vi "Extract Doubles.vi"(4 "error in":errorcluster, 6 "String":string="values: 53k, 42M, separator 37u string as received", 7 "Eng Units?":bool) -> (0 "error out":errorcluster, 3 "Data":dbl[](array[numeric]) format="%_6e")   [LabVIEW 2020]
doc: "Finds all numbers in the given string and puts them into an array as double-precision numbers. All of the following formats are recognized:\n123 1.23 1.23e2 1.23E2\nNo spaces or other characters may appear within the number, but any characters may appear before or after the number.\nThe engineering units convers suffixes k,m,u as 1000, 0.001 and 1e-6 multipliers. Case of the units is not important which means that \"M\" is the same as \"m\" and denotes a 0.001 multiplier.\nModified from examples which did not work, by\nScott Hannahs, <sth@magnet.fsu.edu> NHMFL-FSU, May 2003"
uses:
  <userlib>/_OpenG.lib/array/array.llb/Empty 1D Array (DBL)__ogtk.vi
panel:
  # "This VI takes a string containing multiple numbers and extracts those numbers into an array.  See the Get Info dialog box for more information."
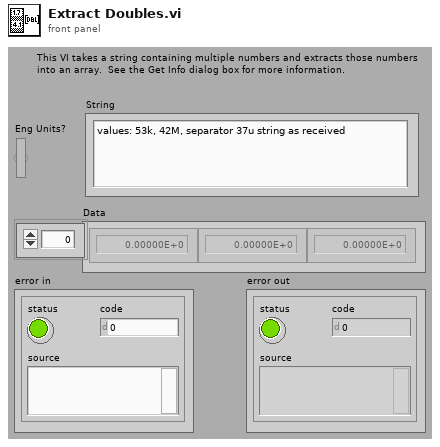
[diagram p1: front panel]
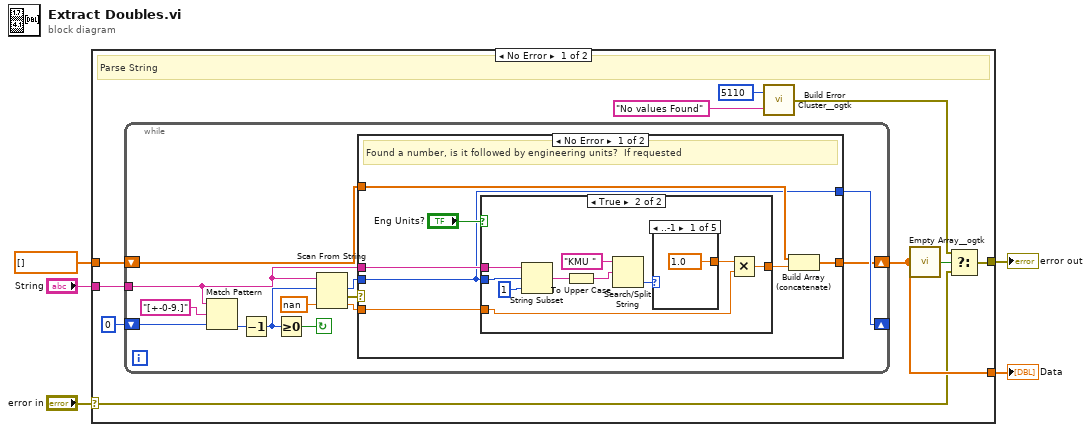
[diagram p0: block diagram]
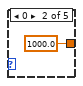
[diagram p3: hidden frame]
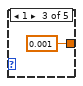
[diagram p4: hidden frame]
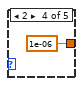
[diagram p5: hidden frame]
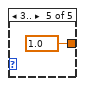
[diagram p6: hidden frame]
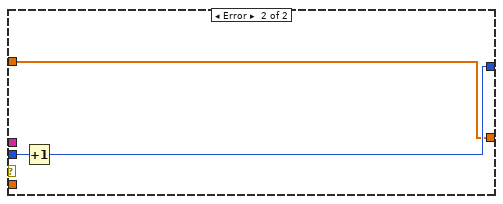
[diagram p7: hidden frame]
diagram:
  n1 = case shown="No Error" "error in" {
    selector: "error in" -> [w11 w56]
    tunnel: "String" -> [w15 _]
    tunnel: dbl[] [] ("Double Precision Array") -> [w14 w55]
    tunnel: [w12 w56] -> w2
    tunnel: [w13 w55] -> w1
    frame No Error {
      # "Parse String"
      n2 = while {
        shift-left: w14 -> [w20]
        shift-right: [w19] -> w13
        tunnel: w15 -> [w17]
        shift-left: u32 0 -> [w27]
        shift-right: [w23] -> _
        stop <- w21 continue-if-true
        n3 = Match Pattern(string=w17, regular expression="[+-0-9.]", offset (0)=w27) -> (offset past match=w26:i32)  [unwired: 3 out]
        n4 = Decrement(x=w26) -> (x-1=w25:i32)
        n5 = Greater Or Equal To 0?(x=w25) -> (x >= 0?=w21:bool)
        n6 = Scan From String(input string=w17, initial scan location=w25, default 1=nan) -> (offset past scan=w22:u32, error out=w16:errorcluster, output 1=w18:dbl)  [unwired: 2 in, 1 out]
        n7 = case shown="No Error" w16 {
          tunnel: [w29 w54] -> w23
          tunnel: w22 -> [w29 w53]
          tunnel: w20 -> [w35 w52]
          tunnel: [w34 w52] -> w19
          tunnel: w18 -> [w32 _]
          tunnel: w17 -> [w30 _]
          frame No Error {
            # "Found a number, is it followed by engineering units?  If requested"
            n8 = case shown="True" "Eng Units?" {
              tunnel: [w36 w41] -> w31
              tunnel: w32 -> [w36 w42]
              tunnel: w30 -> [_ w44]
              tunnel: w29 -> [_ w40]
              frame False {
              }
              frame True {
                n9 = String Subset(string=w44, offset (0)=w40, length (rest)=1 ("length")) -> (substring=w38:string)
                n10 = To Upper Case(1:w38) -> (0:w39:string)
                n11 = Search/Split String(string="KMU ", search string/char (-)=w39) -> (offset of match=w37:i32)  [unwired: 1 in, 2 out]
                n12 = case shown="..-1" w37 {
                  tunnel: [1.0 ("y") 1000.0 ("y") 0.001 ("y") 1e-06 ("y") 1.0 ("y")] -> w43
                  frame ..-1 {
                  }
                  frame 0 {
                  }
                  frame 1 {
                  }
                  frame 2 {
                  }
                  frame 3.. {
                  }
                }
                n13 = Multiply(x=w43, y=w42) -> (x*y=w41:dbl)
              }
            }
            n14 = Build Array (concatenate)(w35, w31) -> (w34:dbl[])
          }
          frame Error {
            n15 = Increment(x=w53) -> (x+1=w54:u32)
          }
        }
      }
      n16 = call <userlib>:"Build Error Cluster__ogtk.vi"("String to Prepend to source (\"\")"="No values Found" ("source"), "code"=5110) -> ("error out"=w8:errorcluster)
      n17 = call-poly <userlib>:"Empty Array__ogtk.vi"("Array"=w13) -> ("Empty Array?"=w10:bool)  [unwired: 8 in]
      n18 = Select(t=w8, s=w10, f=w11) -> (s? t:f=w12:errorcluster)
    }
    frame Error {
      # "Skip Parsing when Error"
    }
  }
  "error out" <- w2
  "Data" <- w1
